vi "BuildSyliineCommCluster.vi"(6 "reply body":string, 7 "Type":string="GET", 8 "reply headers":string, 9 "sent body":string, 10 "sent headers":string, 11 "url":string) -> (0 "Code":i32, 3 "Comm":T1)   [LabVIEW 2016]
uses:
  <userlib>/MicroPython/VIs/SystemLink/SystemLinkHTTPComm.ctl
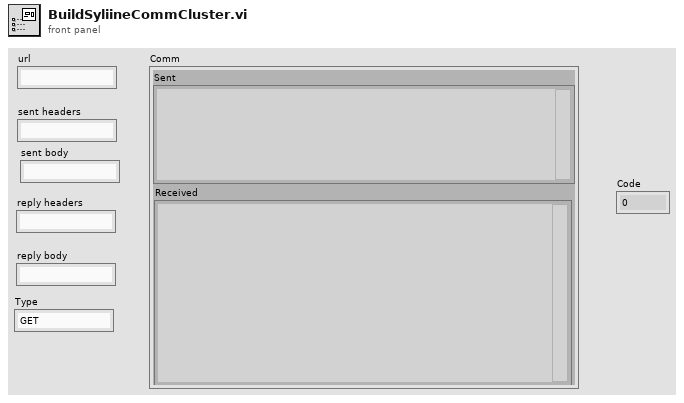
[diagram p1: front panel]
types:
  T1 = typedef "SystemLinkHTTPComm.ctl" = cluster{"url":string, "sent headers":string, "sent body":string, "headers":string, "body":string, "Sent":string, "Received":string}
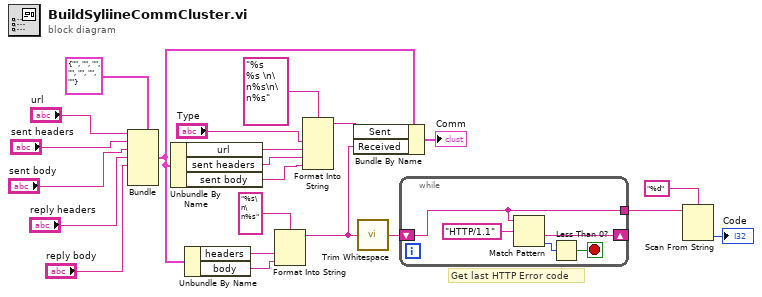
[diagram p0: block diagram]
diagram:
  # "Get last HTTP Error code"
  n1 = Bundle(cluster=T1 {"url"="", "sent headers"="", "sent body"="", "headers"="", "body"="", "Sent"="", "Received"=""} ("Comm"), "url"="url", "sent headers"="sent headers", "sent body"="sent body", "headers"="reply headers", "body"="reply body") -> (w20:T1)  [unwired: 2 in]
  n2 = Unbundle By Name(w20) -> ("url"=w16:string, "sent headers"=w17:string, "sent body"=w7:string)
  n3 = Unbundle By Name(w20) -> ("headers"=w18:string, "body"=w19:string)
  n4 = Format Into String(format string="%s\n\n%s", w18, w19) -> (resulting string=w2:string)  [unwired: 2 in, 1 out]
  n5 = Format Into String(format string="%s %s \n\n%s\n\n%s", "Type", w16, w17, w7) -> (resulting string=w21:string)  [unwired: 2 in, 1 out]
  n6 = Bundle By Name(cluster=w20, "Sent"=w21, "Received"=w2) -> (→"Comm":T1)
  n7 = call <vilib>:"Trim Whitespace.vi"("string"=w2) -> ("trimmed string"=w4:string)  [unwired: 1 in]
  n8 = while {
    shift-right: [w24] -> _
    shift-left: w4 -> [w23]
    tunnel: [w23] -> w5
    stop <- w26 stop-if-true
    n9 = Match Pattern(string=w23, regular expression="HTTP/1.1") -> (after substring=w24:string, offset past match=w25:i32)  [unwired: 1 in, 2 out]
    n10 = Less Than 0?(x=w25) -> (x < 0?=w26:bool)
  }
  n11 = Scan From String(format string="%d", input string=w5) -> (output 1=→"Code":i32)  [unwired: 3 in, 3 out]
